vi "AdminLogInSetNoOfTrials(SubVI).vi"() -> ()   [LabVIEW 2013]
uses:
  <vilib>/addons/database/Connection.llb/DB Tools Open Connec (String).vi
  <vilib>/addons/database/_DB Variant To Data/Database Variant To Data.xnode
  <vilib>/addons/database/NI_Database_API.lvlib
panel:
  in  "Attempts":dbl=5.0
  out "AdminNo.Accepted?":string
  in  "Student Admin No:":string
  in  "Confirm&Back":bool
  # "PLease Enter how many more Attempts for which Student.\n(The default value is 5 trials)"
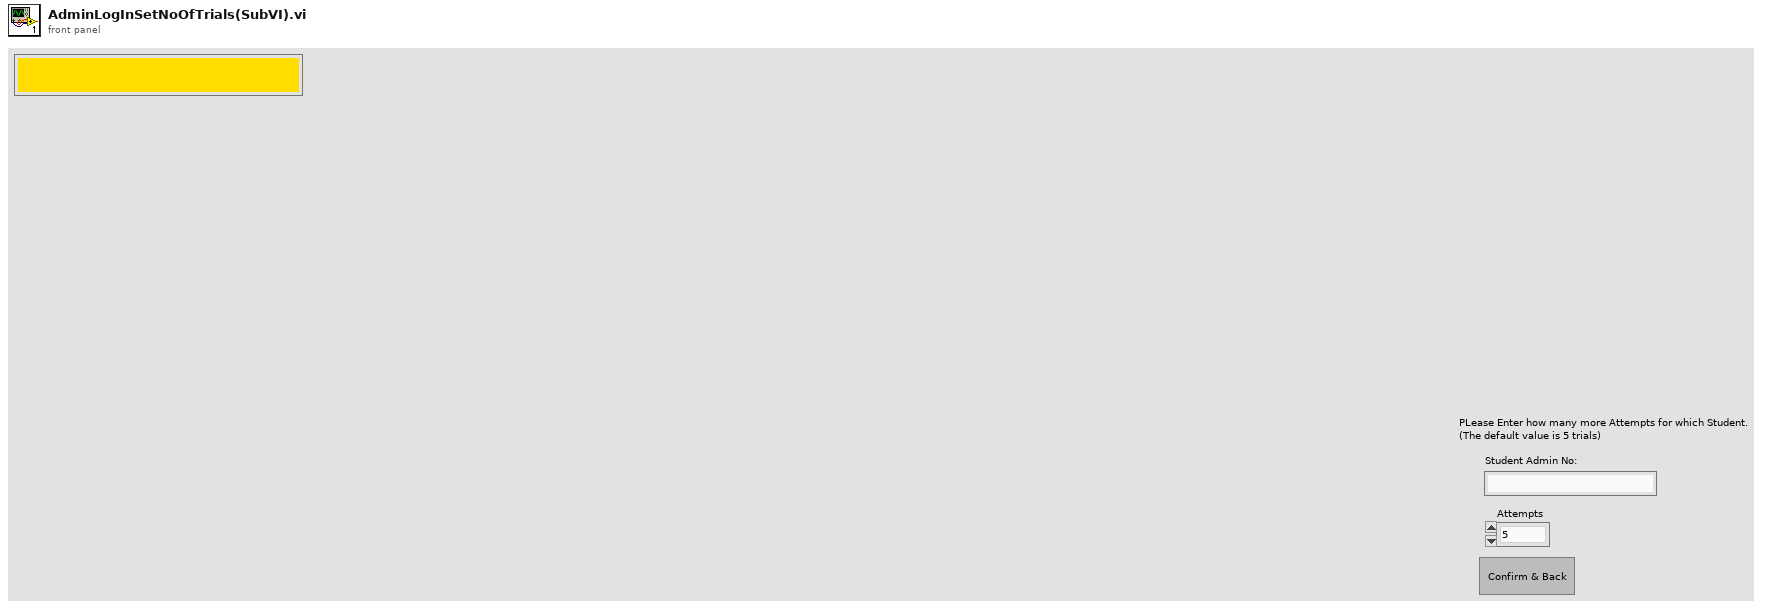
[diagram p1: front panel]
types:
  T1 = typedef "NI_Database_API.lvlib/Conn ObjectReference.ctl" = refnum<k1>
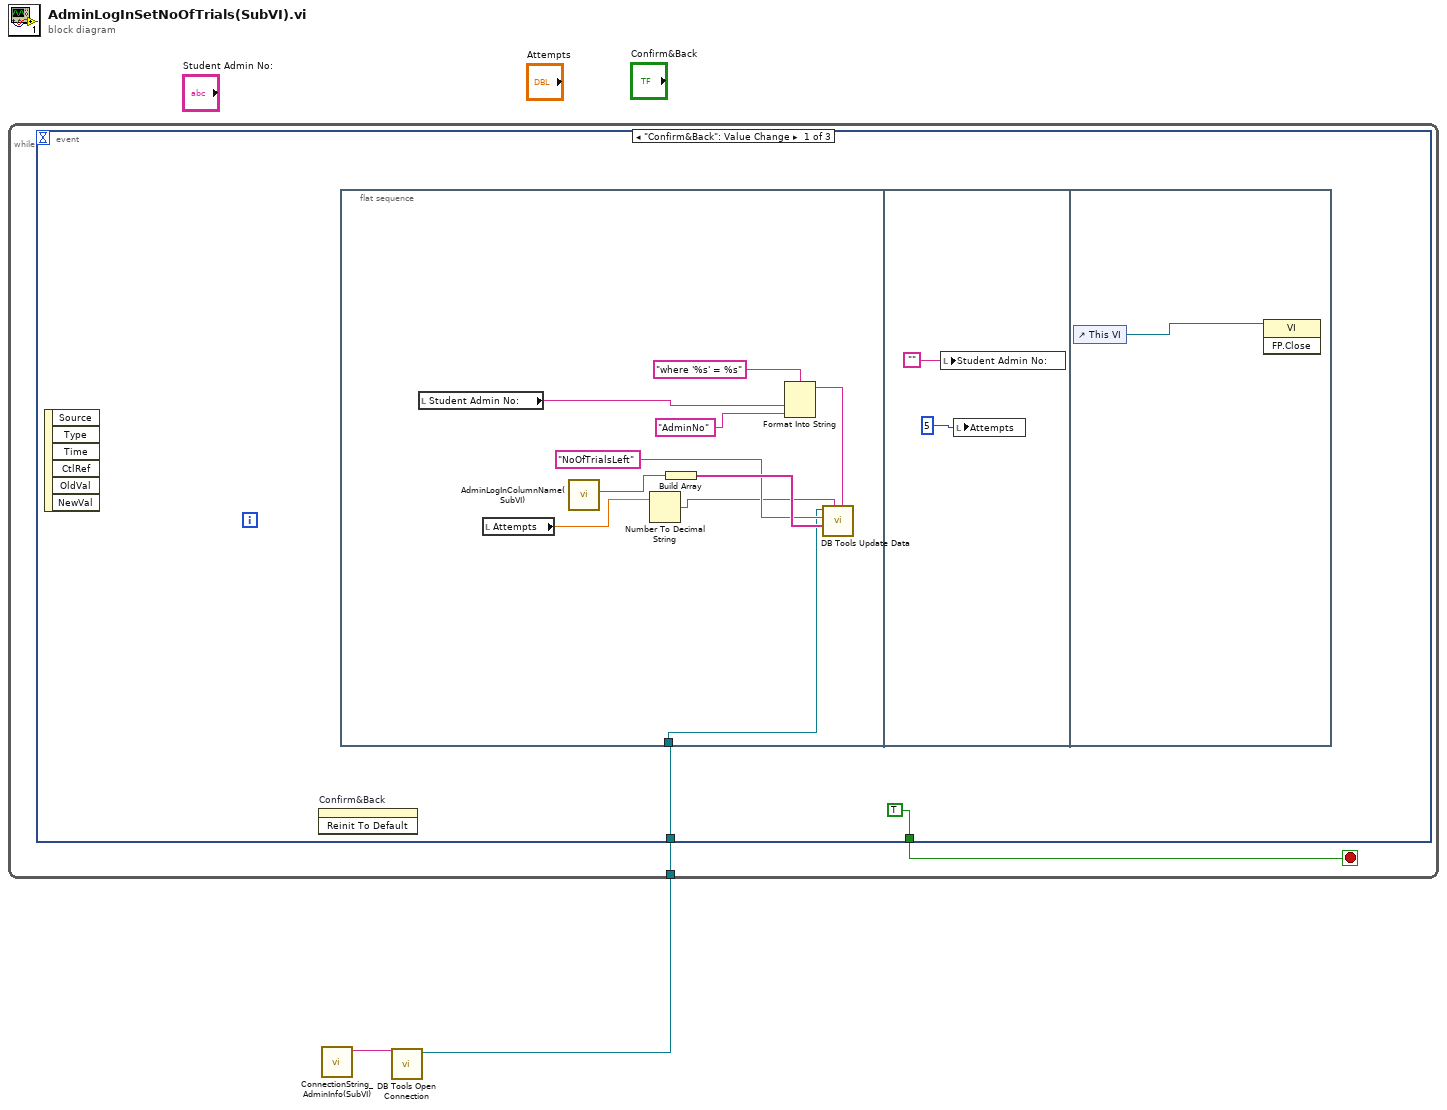
[diagram p0: block diagram]
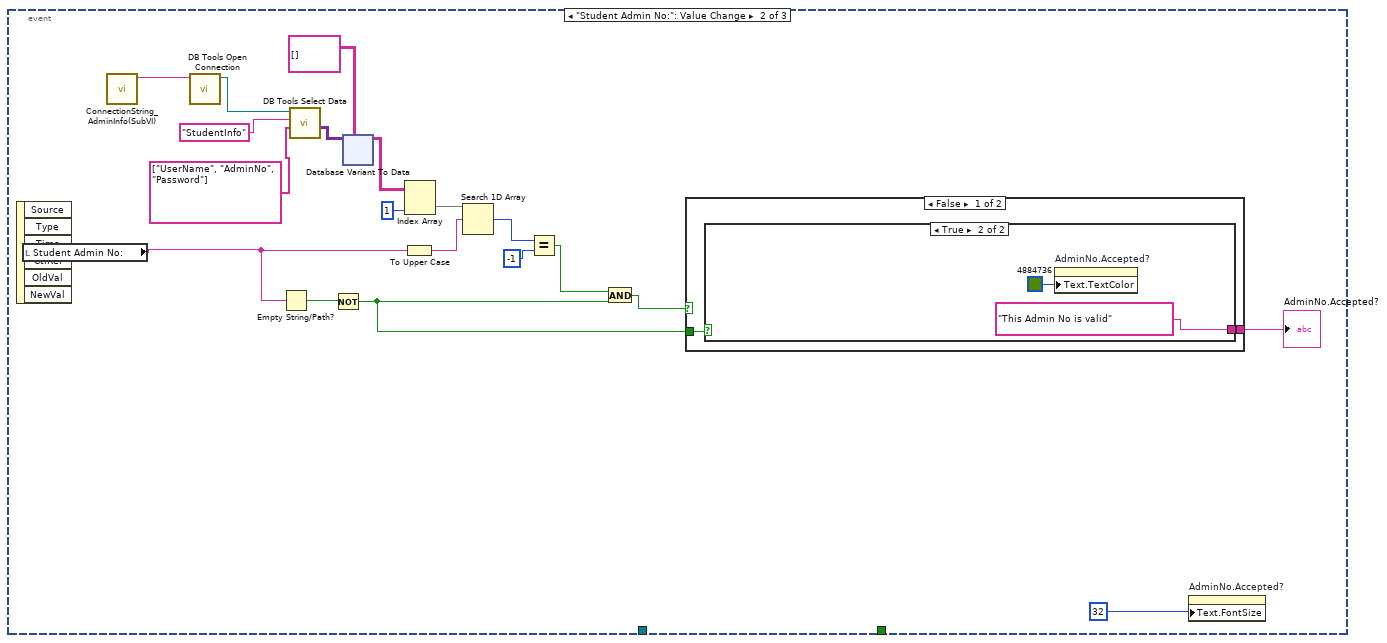
[diagram p2: hidden frame]
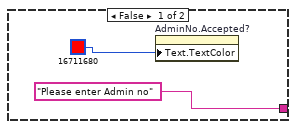
[diagram p3: hidden frame]
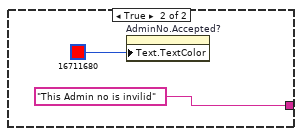
[diagram p4: hidden frame]
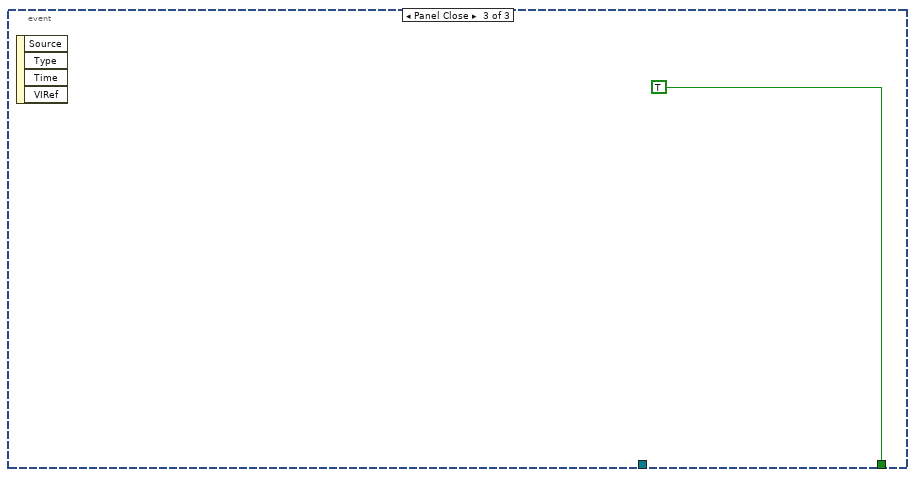
[diagram p5: hidden frame]
diagram:
  n1 = call "ConnectionString_AdminInfo(SubVI).vi"() -> ("ConnectionString"=w2:string)  [unwired: 11 in]
  n2 = call-poly <vilib>:"DB Tools Open Connection.vi"("connection information"=w2) -> ("connection reference"=w1:T1)  [unwired: 7 in, 1 out]
  n3 = while {
    tunnel: w1 -> [w3]
    stop <- w4 stop-if-true
    n4 = event shown="[0] \"Confirm&Back\": Value Change" {
      selector: _ -> [_ _ _]
      dyn-events: _ -> [_ _ _]
      timeout: _ -> [_ _ _]
      tunnel: [TRUE _ TRUE] -> w4
      tunnel: w3 -> [w5 _ _]
      event "Confirm&Back": Value Change {
        n5 = event-data() -> ()  [unwired: 1 in, 6 out]
        n6 = invoke on="Confirm&Back" class="Bool (strict)" method="Reinit To Default"() -> ()  [unwired: 3 in, 3 out]
        n7 = flat-sequence {
          tunnel: w5 -> [w9]
          frame #0 {
            n8 = local read "Student Admin No:"() -> (w8:string)
            n9 = local read "Attempts"() -> (w7:dbl)
            n10 = call "AdminLogInColumnName(SubVI).vi"() -> ("Path for Score Table"=w10:string)  [unwired: 11 in]
            n11 = Number To Decimal String(number=w7) -> (decimal integer string=w11:string)  [unwired: 1 in]
            n12 = Build Array(w10) -> (w13:string[])
            n13 = Format Into String(format string="where '%s' = %s", w8, "AdminNo") -> (resulting string=w16:string)  [unwired: 2 in, 1 out]
            n14 = call <vilib>:"DB Tools Update Data.vi"("condition"=w16, "data"=w11, "columns"=w13, "table"="NoOfTrialsLeft", "connection reference"=w9) -> ()  [unwired: 5 in, 2 out]
          }
          frame #1 {
            n15 = local write "Student Admin No:"("") -> ()
            n16 = local write "Attempts"(5) -> ()
          }
          frame #2 {
            n17 = control-ref of="This VI"() -> (w19:refnum<vi>)
            n18 = invoke class="VI" method="FP.Close"(reference=w19) -> ()  [unwired: 2 in, 3 out]
          }
        }
      }
      event "Student Admin No:": Value Change {
        n19 = event-data() -> ()  [unwired: 1 in, 6 out]
        n20 = local read "Student Admin No:"() -> (w21:string)
        n21 = call "ConnectionString_AdminInfo(SubVI).vi"() -> ("ConnectionString"=w36:string)  [unwired: 11 in]
        n22 = call-poly <vilib>:"DB Tools Open Connection.vi"("connection information"=w36) -> ("connection reference"=w37:T1)  [unwired: 7 in, 1 out]
        n23 = Empty String/Path?(string/path=w21) -> (empty?=w31:bool)
        n24 = call <vilib>:"DB Tools Select Data.vi"("columns"=string[] ["UserName", "AdminNo", "Password"], "table"="StudentInfo", "connection reference"=w37) -> ("data"=w24:variant[][])  [unwired: 3 in, 2 out]
        n25 = Not(x=w31) -> (.not. x?=w33:bool)
        n26 = xnode "Database Variant To Data"("database variant"=w24, "type"=string[][] []) -> ("data"=w25:string[][])  [unwired: 1 in, 1 out]
        n27 = To Upper Case(1:w21) -> (0:w28:string)
        n28 = Index Array(array=w25, index (col)=1) -> (element=w27:string[])  [unwired: 1 in]
        n29 = Search 1D Array(1D array=w27, element=w28) -> (index of element=w29:i32)  [unwired: 1 in]
        n30 = Equal?(x=w29, y=-1) -> (x = y?=w32:bool)
        n31 = And(x=w32, y=w33) -> (x .and. y?=w38:bool)
        n32 = case shown="False" w38 {
          tunnel: w33 -> [w39 _]
          tunnel: [w40 "This Admin no is invilid"] -> w34
          frame False {
            n33 = case shown="True" w39 {
              tunnel: ["Please enter Admin no" "This Admin No is valid"] -> w40
              frame False {
                n34 = property on="AdminNo.Accepted?" class="Str"("Text.TextColor"=u32 16711680) -> ()  [unwired: 2 in, 2 out]
              }
              frame True {
                n35 = property on="AdminNo.Accepted?" class="Str"("Text.TextColor"=u32 4884736) -> ()  [unwired: 2 in, 2 out]
              }
            }
          }
          frame True {
            n36 = property on="AdminNo.Accepted?" class="Str"("Text.TextColor"=u32 16711680) -> ()  [unwired: 2 in, 2 out]
          }
        }
        "AdminNo.Accepted?" <- w34
        n37 = property on="AdminNo.Accepted?" class="Str"("Text.FontSize"=32) -> ()  [unwired: 2 in, 2 out]
      }
      event Panel Close {
        n38 = event-data() -> ()  [unwired: 1 in, 4 out]
      }
    }
  }
